vi "RPC Fast Server (test).vi"() -> ()   [LabVIEW 2020]
uses:
  External/JSON-RPC/Classes/Server/Add Response (Result from Request).vi
  External/JSON-RPC/Classes/Server/Add Response (Server Error from Request).vi
  External/JSON-RPC/Classes/Server/Add Response (Internal Error from Request).vi
  External/JSON-RPC/Classes/Server/Send Request (Sync).vi
  External/JSON-RPC/Classes/Server/JSONRPC Server.lvclass
  Realization/RPC.lvlib
panel:
  out "request":string
  out "response":string
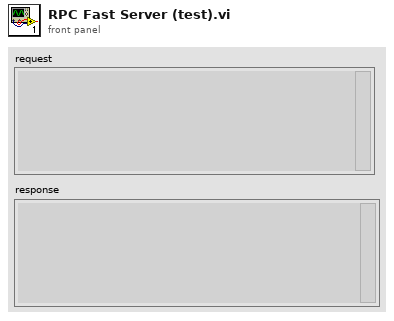
[diagram p1: front panel]
types:
  T1 = enum16{"Standard", "Buffered", "CRLF", "Immediate"}
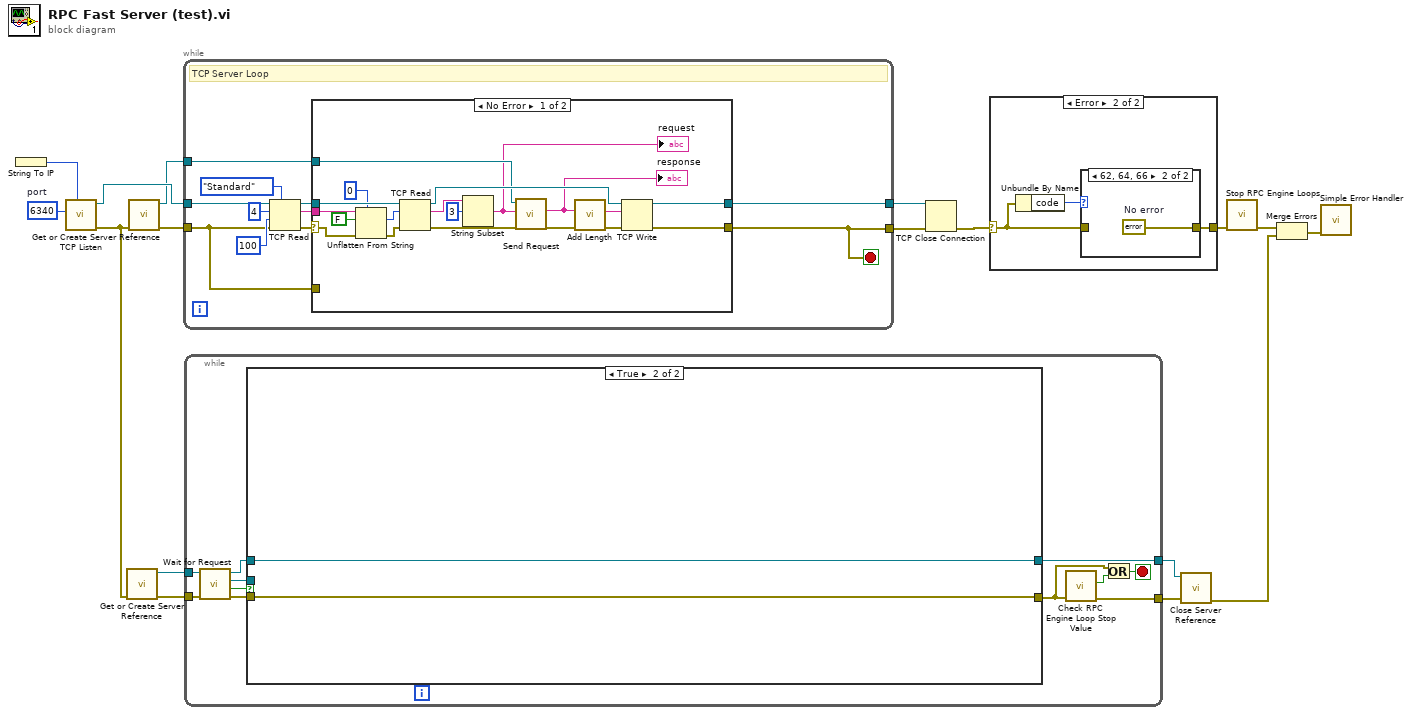
[diagram p0: block diagram]
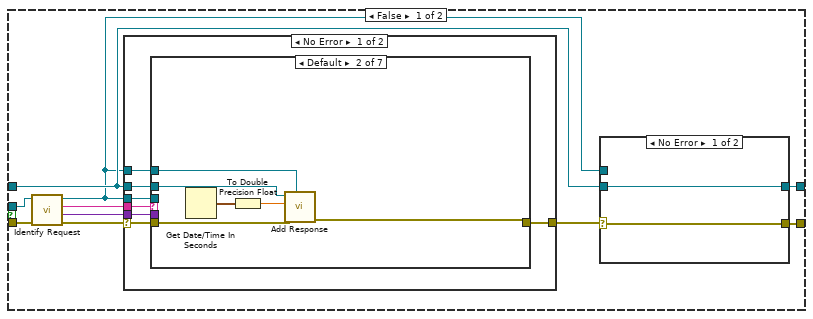
[diagram p2: hidden frame]
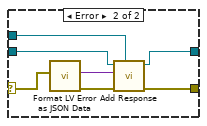
[diagram p3: hidden frame]
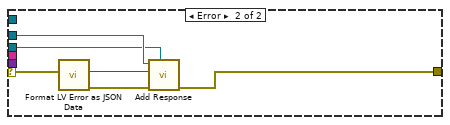
[diagram p10: hidden frame]
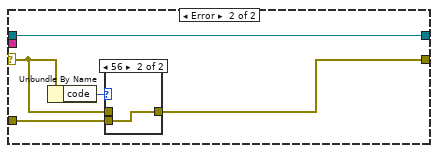
[diagram p13: hidden frame]
diagram:
  w15 = u16 6340  # port
  n1 = String To IP() -> (0:w14:u32)  [unwired: 1 in]
  n2 = call <vilib>:"TCP Listen.vi"("net address"=w14, "port"=w15) -> ("error out"=w3:errorcluster, "connection ID"=w12:refnum<k5>)  [unwired: 5 in, 3 out]
  n3 = call "Get or Create Server Reference.vi"("error in (no error)"=w3) -> ("error out"=w8:errorcluster, "Server Out"=w1:refnum<class "JSONRPC Server.lvclass">)  [unwired: 9 in]
  n4 = call "Get or Create Server Reference.vi"("error in (no error)"=w3) -> ("error out"=w11:errorcluster, "Server Out"=w10:refnum<class "JSONRPC Server.lvclass">)  [unwired: 9 in]
  n5 = while {
    tunnel: [w18] -> w16
    tunnel: [w25] -> w17
    tunnel: w12 -> [w21]
    tunnel: w11 -> [w22]
    tunnel: w10 -> [w19]
    stop <- w18 stop-if-true
    # "TCP Server Loop"
    n6 = TCP Read(connection ID=w21, bytes to read=4, error in (no error)=w22, 7:T1."Standard" ("mode (standard)"), 9:100 ("timeout ms (25000)")) -> (connection ID out=w26:refnum<k5>, data out=w20:string, error out=w24:errorcluster)
    n7 = case shown="No Error" w24 {
      selector: w24 -> [w37 w51]
      tunnel: [w45 w49] -> w18
      tunnel: w22 -> [_ w50]
      tunnel: [w46 w48] -> w25
      tunnel: w26 -> [w47 w48]
      tunnel: w20 -> [w33 _]
      tunnel: w19 -> [w42 _]
      frame No Error {
        n8 = Unflatten From String(type=0, binary string=w33, data includes array or string size? (T)=FALSE, error in (no error)=w37) -> (value=w34:i32, error out=w36:errorcluster)  [unwired: 1 in, 1 out]
        n9 = TCP Read(connection ID=w47, bytes to read=w34, error in (no error)=w36) -> (connection ID out=w44:refnum<k5>, data out=w32:string, error out=w43:errorcluster)  [unwired: 2 out]
        n10 = String Subset(string=w32, offset (0)=3) -> (substring=w31:string)  [unwired: 1 in]
        "request" <- w31
        n11 = call-poly "Send Request.vi"("error in (no error)"=w43, "JSON Request String"=w31, "JSONRPC Server in"=w42) -> ("error out"=w41:errorcluster, "JSON Response String"=w29:string)  [unwired: 6 in, 1 out]
        "response" <- w29
        n12 = call "Add Length.vi"("error in (no error)"=w41, "JSON Response String in"=w29) -> ("error out"=w40:errorcluster, "JSON Response String out"=w39:string)  [unwired: 8 in]
        n13 = TCP Write(connection ID=w44, data in=w39, error in (no error)=w40) -> (connection ID out=w46:refnum<k5>, error out=w45:errorcluster)  [unwired: 1 in, 1 out]
      }
      frame Error {
        n14 = Unbundle By Name(w51) -> ("code"=w52:i32)
        n15 = case shown="56" w52 {
          tunnel: w51 -> [w53 _]
          tunnel: w50 -> [_ w54]
          tunnel: [w53 w54] -> w49
          frame Default {
          }
          frame 56 {
          }
        }
      }
    }
  }
  n16 = while {
    tunnel: w8 -> [w65]
    tunnel: w1 -> [w64]
    tunnel: [w59] -> w7
    tunnel: [w58] -> w6
    stop <- w55 stop-if-true
    n17 = call "Wait for Request.vi"("error in (no error)"=w65, "Server in"=w64) -> ("error out"=w63:errorcluster, "timed out?"=w60:bool, "Request"=w62:refnum<class "Request.lvclass">, "Server out"=w61:refnum<class "JSONRPC Server.lvclass">)  [unwired: 6 in]
    n18 = case shown="True" w60 {
      tunnel: w63 -> [w69 w111]
      tunnel: w62 -> [w75 _]
      tunnel: w61 -> [w67 w110]
      tunnel: [w72 w111] -> w56
      tunnel: [w71 w110] -> w58
      frame False {
        n19 = call "Identify Request.vi"("error in (no error)"=w69, "Request in"=w75) -> ("error out"=w70:errorcluster, "params"=w74:variant, "method"=w68:string, "Request out"=w66:refnum<class "Request.lvclass">)  [unwired: 5 in, 1 out]
        n20 = case shown="No Error" w70 {
          selector: w70 -> [w89 w109]
          tunnel: w74 -> [w86 _]
          tunnel: w67 -> [w91 w107]
          tunnel: w66 -> [w90 w106]
          tunnel: [w88 w104] -> w73
          tunnel: w68 -> [w87 _]
          tunnel: w66 -> [w85 _]
          frame No Error {
            n21 = case shown="Default" w87 {
              tunnel: w91 -> [_ w97 _ _ _ _ _]
              tunnel: w90 -> [_ _ _ _ _ _ _]
              tunnel: w89 -> [w92 w98 w99 w100 w101 w102 w103]
              tunnel: [w92 w95 w99 w100 w101 w102 w103] -> w88
              tunnel: w86 -> [_ _ _ _ _ _ _]
              tunnel: w85 -> [_ w96 _ _ _ _ _]
              frame "rpc_server_init" {
              }
              frame Default {
                n22 = Get Date/Time In Seconds() -> (seconds since 1Jan1904=w93:timestamp)
                n23 = To Double Precision Float(number=w93) -> (double precision float=w94:dbl)
                n24 = call-poly "Add Response.vi"("Request"=w96, "error in (no error)"=w98, "JSON Value in"=w94, "Server in"=w97) -> ("error out"=w95:errorcluster)  [unwired: 5 in, 2 out]
              }
              frame "rpc_server_dispatch" {
              }
              frame "rpc_server_launch_module" {
              }
              frame "rpc_server_shutdown_module" {
              }
              frame "rpc_server_broadcast" {
              }
              frame "rpc_server_shutdown" {
              }
            }
          }
          frame Error {
            n25 = call "Format LV Error as JSON Data.vi"("error in"=w109) -> ("error out"=w108:errorcluster, "Error Value out"=w105:variant)  [unwired: 9 in]
            n26 = call-poly "Add Response.vi"("Request"=w106, "error in (no error)"=w108, "data"=w105, "Server in"=w107) -> ("error out"=w104:errorcluster)  [unwired: 5 in, 2 out]
          }
        }
        n27 = case shown="No Error" w73 {
          selector: w73 -> [w77 w82]
          tunnel: [w77 w81] -> w72
          tunnel: w67 -> [w76 w79]
          tunnel: [w76 w80] -> w71
          tunnel: w66 -> [_ w78]
          frame No Error {
          }
          frame Error {
            n28 = call "Format LV Error as JSON Data.vi"("error in"=w82) -> ("error out"=w84:errorcluster, "Error Value out"=w83:variant)  [unwired: 9 in]
            n29 = call-poly "Add Response.vi"("Request"=w78, "error in (no error)"=w84, "data"=w83, "Server in"=w79) -> ("error out"=w81:errorcluster, "Server out"=w80:refnum<class "JSONRPC Server.lvclass">)  [unwired: 5 in, 1 out]
          }
        }
      }
      frame True {
      }
    }
    n30 = call "Check RPC Engine Loop Stop Value.vi"("error in (no error)"=w56) -> ("error out"=w59:errorcluster, "stopped?"=w57:bool)  [unwired: 9 in]
    n31 = Or(x=w56, y=w57) -> (x .or. y?=w55:bool)
  }
  n32 = TCP Close Connection(connection ID=w17, error in (no error)=w16) -> (error out=w13:errorcluster)  [unwired: 2 out]
  n33 = case shown="Error" w13 {
    selector: w13 -> [w112 w114]
    tunnel: [w112 w113] -> w9
    frame No Error {
    }
    frame Error {
      n34 = Unbundle By Name(w114) -> ("code"=w115:i32)
      n35 = case shown="62, 64, 66" w115 {
        tunnel: w114 -> [w116 _]
        tunnel: [w116 w117] -> w113
        frame Default {
        }
        frame 62, 64, 66 {
          w117 = errorcluster {"status"=FALSE, "code"=0, "source"=""}  # No error
        }
      }
    }
  }
  n36 = call "Close Server Reference.vi"("error in (no error)"=w7, "Server in"=w6) -> ("error out"=w2:errorcluster)  [unwired: 9 in]
  n37 = call "Stop RPC Engine Loops.vi"("error in (no error)"=w9) -> ("error out"=w5:errorcluster)  [unwired: 10 in]
  n38 = Merge Errors(w5, w2) -> (w4:errorcluster)
  n39 = call <vilib>:"Simple Error Handler.vi"("error in (no error)"=w4) -> ()  [unwired: 1 in, 8 out]
